vi "BRig_RT__Case_Exp__State_WrongOrTimeout_Pre__v10.vi"(0 "input_dataCurrent":u16[](array[numeric]), 5 "input_WorTO":bool, 7 "input_dataBlock":u16[][](array[numeric]), 9 "input_dataTrial":u16[][](array[numeric]), 11 "input_dataExp":u16[](array[numeric])) -> (1 "output_BTPR":bool, 2 "output_T2R":bool, 3 "output_T2R_or_BTPR":u16, 4 "output_dataCurrent":u16[](array[numeric]), 8 "output_dataBlock":u16[][](array[numeric]), 10 "output_dataTrial":u16[][](array[numeric]), 12 "output_BTPRavg":dbl, 13 "output_T2Ravg":dbl, 14 "output_R(F)_or_L(T)":bool, 15 "output_haveNewAvg":bool)   [LabVIEW 2014]
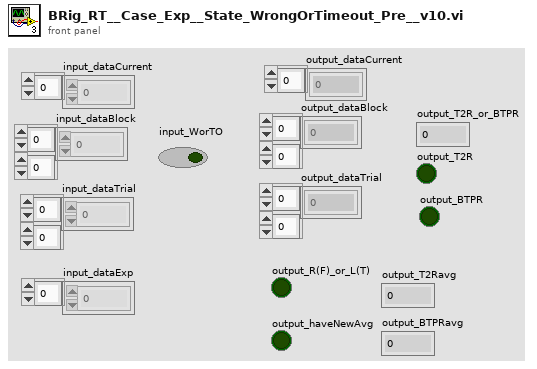
[diagram p1: front panel]
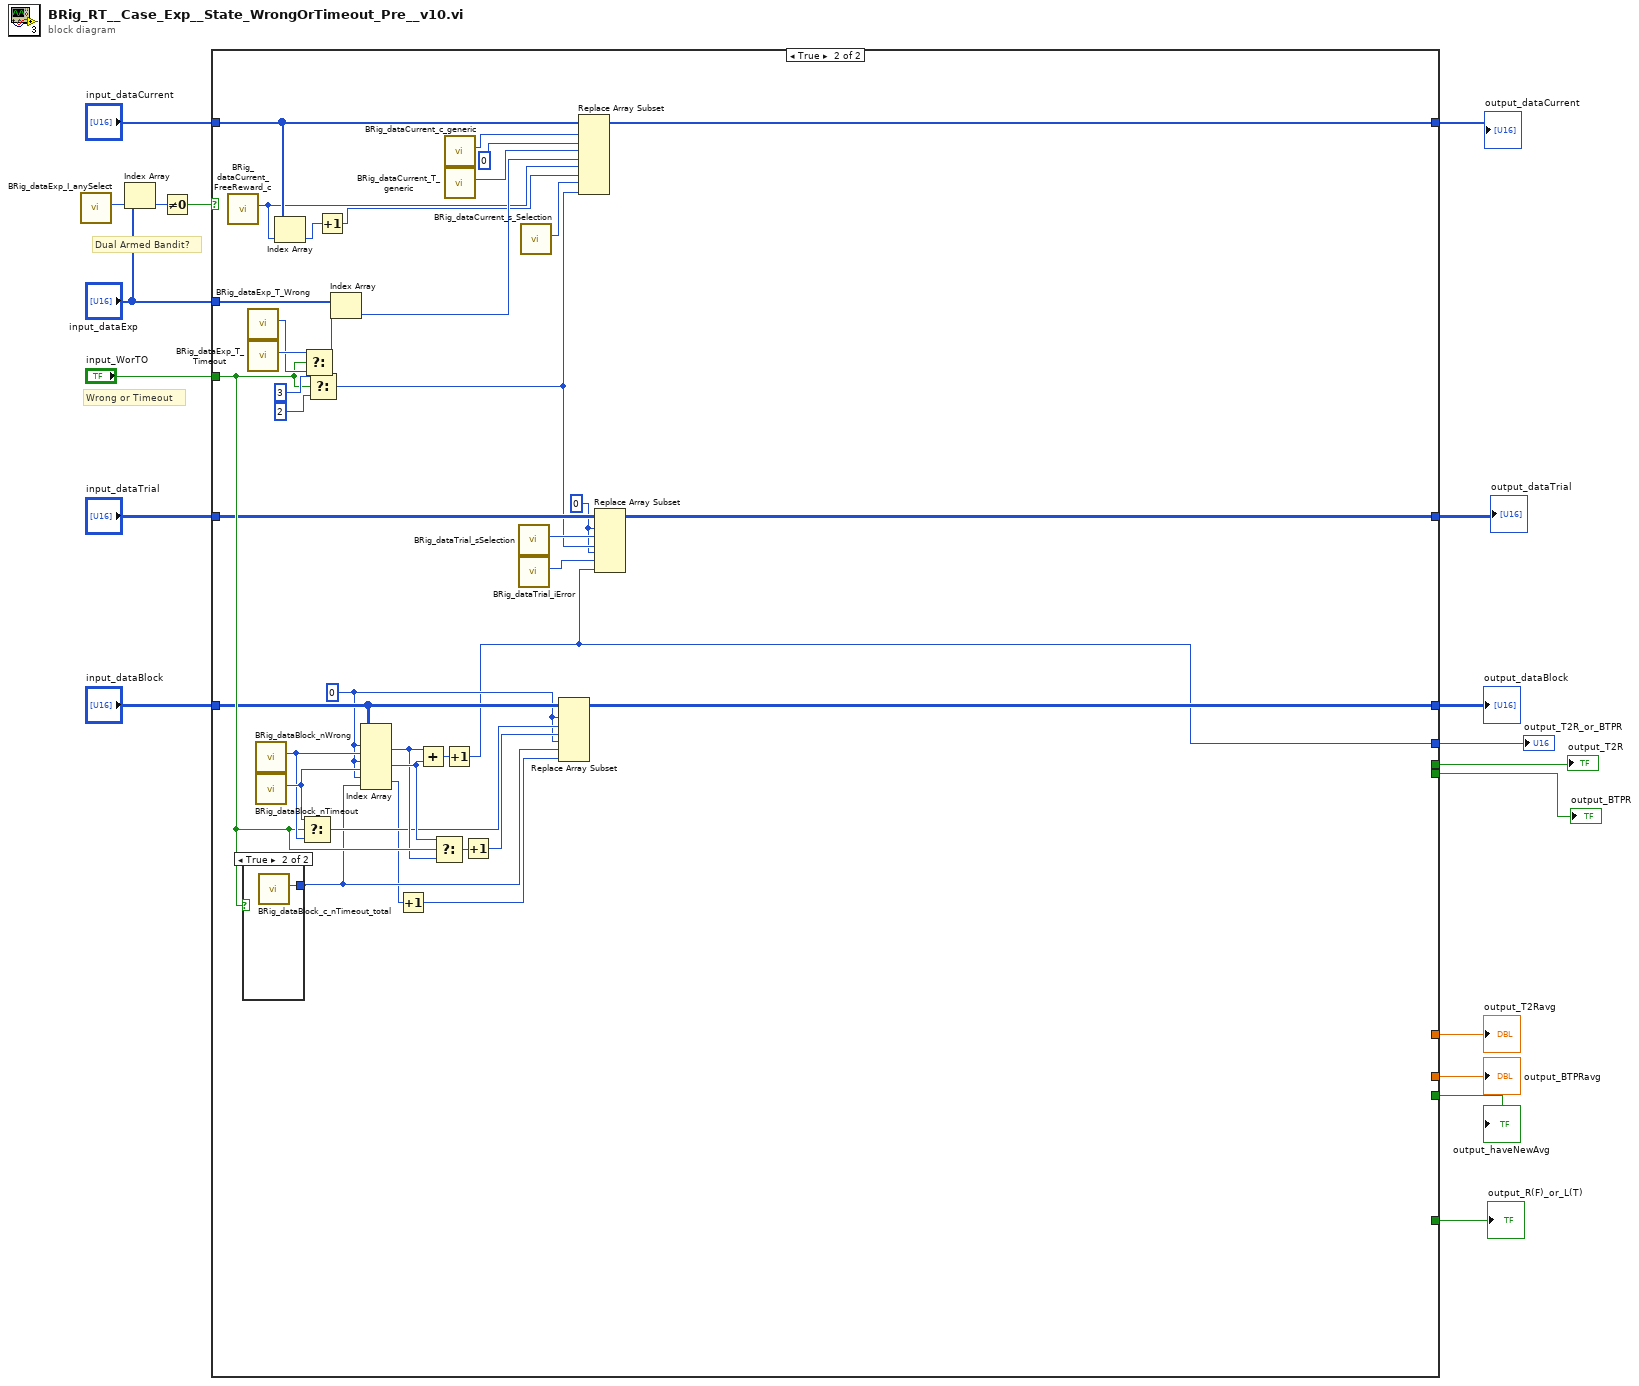
[diagram p0: block diagram]
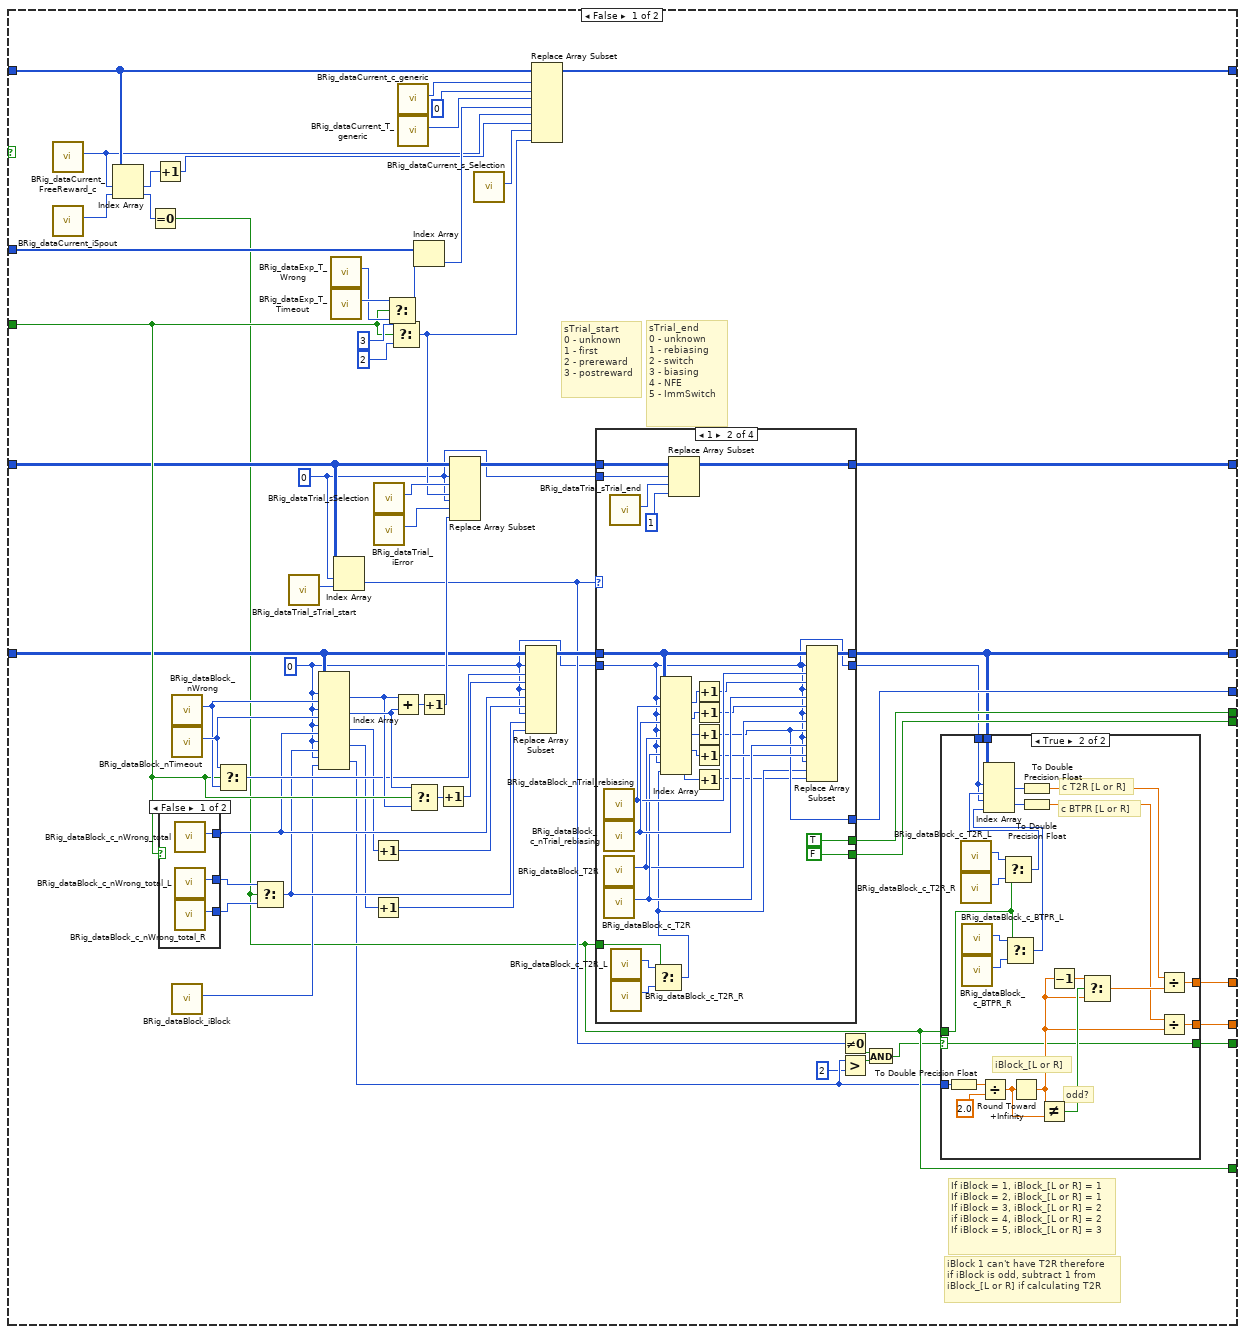
[diagram p2: hidden frame]
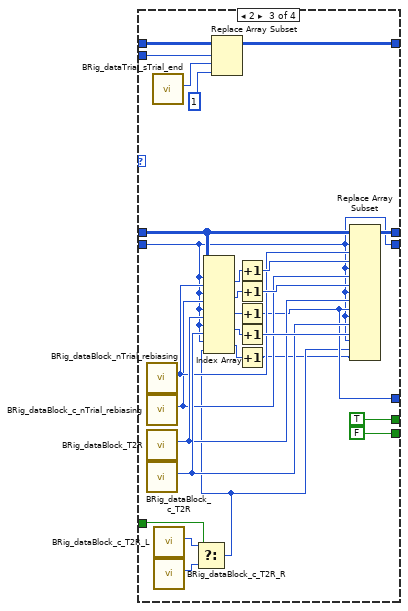
[diagram p5: hidden frame]
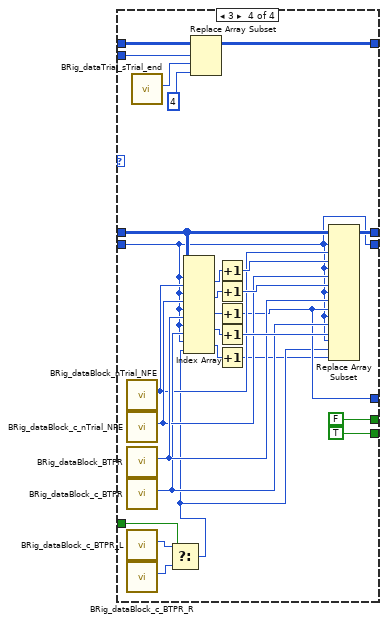
[diagram p6: hidden frame]
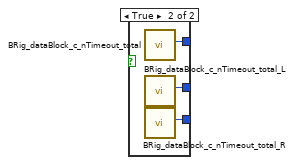
[diagram p7: hidden frame]
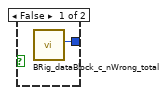
[diagram p8: hidden frame]
diagram:
  # "Wrong or Timeout"
  # "Dual Armed Bandit?"
  n1 = call "BRig_dataExp_I_anySelect.vi"() -> ("output_I_anySelect"=w5:i32)  [unwired: 11 in]
  n2 = Index Array(array="input_dataExp", index=w5) -> (element=w4:u16)
  n3 = Not Equal To 0?(x=w4) -> (x != 0?=w2:bool)
  n4 = case shown="True" w2 {
    tunnel: [w81 w236] -> w18
    tunnel: "input_dataCurrent" -> [w77 w232]
    tunnel: "input_dataExp" -> [w76 w231]
    tunnel: "input_WorTO" -> [w61 w219]
    tunnel: "input_dataBlock" -> [w57 w215]
    tunnel: "input_dataTrial" -> [w47 w209]
    tunnel: [w44 w202] -> w1
    tunnel: [w38 w199] -> w13
    tunnel: [w37 _] -> w12
    tunnel: [w36 _] -> w11
    tunnel: [w29 _] -> w10
    tunnel: [w28 w201] -> w9
    tunnel: [w26 _] -> w8
    tunnel: [w25 _] -> w7
    tunnel: [w24 _] -> w6
    frame False {
      w32 = 0
      w33 = 0
      # "iBlock 1 can't have T2R therefore\nif iBlock is odd, subtract 1 from\niBlock_[L or R] if calculating T2R"
      # "If iBlock = 1, iBlock_[L or R] = 1\nIf iBlock = 2, iBlock_[L or R] = 1\nIf iBlock = 3, iBlock_[L or R] = 2\nif iBlock = 4, iBlock_[L or R] = 2\nIf iBlock = 5, iBlock_[L or R] = 3"
      # "sTrial_end\n0 - unknown\n1 - rebiasing\n2 - switch\n3 - biasing\n4 - NFE\n5 - ImmSwitch"
      # "sTrial_start\n0 - unknown\n1 - first\n2 - prereward\n3 - postreward"
      n5 = call "BRig_dataCurrent_FreeReward_c.vi"() -> ("output_FreeReward_c"=w42:i32)  [unwired: 11 in]
      n6 = call "BRig_dataCurrent_iSpout.vi"() -> ("output_iSpout"=w31:i32)  [unwired: 11 in]
      n7 = Index Array(array=w77, index #1=w42, index #2=w31) -> (element #1=w43:u16, element #2=w30:u16)
      n8 = Equal To 0?(x=w30) -> (x = 0?=w29:bool)
      n9 = Increment(x=w43) -> (x+1=w41:u16)
      n10 = case shown="False" w61 {
        tunnel: [w195 w198] -> w54
        tunnel: [w194 w197] -> w67
        tunnel: [w193 w196] -> w66
        frame False {
          n11 = call "BRig_dataBlock_c_nWrong_total.vi"() -> ("output_c_nWrong_total"=w195:i32)  [unwired: 11 in]
          n12 = call "BRig_dataBlock_c_nWrong_total_L.vi"() -> ("output_c_nWrong_total_L"=w194:i32)  [unwired: 11 in]
          n13 = call "BRig_dataBlock_c_nWrong_total_R.vi"() -> ("output_c_nWrong_total_R"=w193:i32)  [unwired: 11 in]
        }
        frame True {
          n14 = call "BRig_dataBlock_c_nTimeout_total.vi"() -> ("output_c_nTimeout_total"=w198:i32)  [unwired: 11 in]
          n15 = call "BRig_dataBlock_c_nTimeout_total_L.vi"() -> ("output_c_nTimeout_total_L"=w197:i32)  [unwired: 11 in]
          n16 = call "BRig_dataBlock_c_nTimeout_total_R.vi"() -> ("output_c_nTimeout_total_R"=w196:i32)  [unwired: 11 in]
        }
      }
      n17 = call "BRig_dataBlock_nWrong.vi"() -> ("output_nWrong"=w62:i32)  [unwired: 11 in]
      n18 = call "BRig_dataBlock_nTimeout.vi"() -> ("output_nTimeout"=w63:i32)  [unwired: 11 in]
      n19 = call "BRig_dataBlock_iBlock.vi"() -> ("output_iBlock"=w35:i32)  [unwired: 11 in]
      n20 = Select(t=w63, s=w61, f=w62) -> (s? t:f=w56:i32)
      n21 = Select(t=w67, s=w29, f=w66) -> (s? t:f=w53:i32)
      n22 = call "BRig_dataTrial_sTrial_start.vi"() -> ("output_sTrial_start"=w48:i32)  [unwired: 11 in]
      n23 = Index Array(array=w57, index (row) #1=w32, index (col) #1=w62, index (row) #2=w32, index (col) #2=w63, index (row) #3=w32, index (col) #3=w54, index (row) #4=w32, index (col) #4=w53, index (row) #5=w32, index (col) #5=w35) -> (element #1=w59:u16, element #2=w60:u16, element #3=w52:u16, element #4=w51:u16, element #5=w23:u16)
      n24 = call "BRig_dataExp_T_Wrong.vi"() -> ("output_T_Wrong"=w73:i32)  [unwired: 11 in]
      n25 = call "BRig_dataExp_T_Timeout.vi"() -> ("output_T_Timeout"=w74:i32)  [unwired: 11 in]
      n26 = Index Array(array=w47, index (row)=w33, index (col)=w48) -> (element=w34:u16)
      n27 = Increment(x=w52) -> (x+1=w50:u16)
      n28 = Increment(x=w51) -> (x+1=w49:u16)
      n29 = call "BRig_dataTrial_sSelection.vi"() -> ("output_sSelection"=w69:i32)  [unwired: 11 in]
      n30 = call "BRig_dataTrial_iError.vi"() -> ("output_iError"=w68:i32)  [unwired: 11 in]
      n31 = Select(t=w74, s=w61, f=w73) -> (s? t:f=w75:i32)
      n32 = Select(t=u16 3 ("new element/subarray"), s=w61, f=u16 2 ("new element/subarray")) -> (s? t:f=w39:u16)
      n33 = Add(x=w59, y=w60) -> (x+y=w65:u16)
      n34 = call "BRig_dataCurrent_c_generic.vi"() -> ("output_count_generic"=w80:i32)  [unwired: 11 in]
      n35 = call "BRig_dataCurrent_T_generic.vi"() -> ("output_T_generic"=w79:i32)  [unwired: 11 in]
      n36 = Select(t=w60, s=w61, f=w59) -> (s? t:f=w58:u16)
      n37 = Index Array(array=w76, index=w75) -> (element=w72:u16)
      n38 = Increment(x=w65) -> (x+1=w64:u16)
      n39 = Increment(x=w58) -> (x+1=w55:u16)
      n40 = Replace Array Subset(array=w47, new element #1=w39, index (row) #1=w33, index (col) #1=w69, new element #2=w64, index (row) #2=w33, index (col) #2=w68) -> (w46:u16[][])
      n41 = call "BRig_dataCurrent_s_Selection.vi"() -> ("output_s_Selection"=w40:i32)  [unwired: 11 in]
      n42 = Replace Array Subset(array=w57, new element #1=w55, index (row) #1=w32, index (col) #1=w56, new element #2=w50, index (row) #2=w32, index (col) #2=w54, new element #3=w49, index (row) #3=w32, index (col) #3=w53) -> (w45:u16[][])
      n43 = Replace Array Subset(array=w77, new element #1=u16 0 ("new element/subarray"), index #1=w80, new element #2=w72, index #2=w79, new element #3=w41, index #3=w42, new element #4=w39, index #4=w40) -> (w81:u16[])
      n44 = case shown="1" w34 {
        tunnel: w46 -> [w108 w136 w164 w192]
        tunnel: w33 -> [_ w134 w162 w190]
        tunnel: [w108 w135 w163 w191] -> w44
        tunnel: w45 -> [w107 w125 w148 w180]
        tunnel: [w107 w124 w147 w179] -> w28
        tunnel: w32 -> [w106 w109 w137 w165]
        tunnel: [_ w116 w146 w172] -> w38
        tunnel: [_ TRUE TRUE FALSE] -> w37
        tunnel: [_ FALSE FALSE TRUE] -> w36
        tunnel: w29 -> [_ w115 w139 w171]
        tunnel: [w106 w109 w137 w165] -> w27
        frame 0, Default {
        }
        frame 1 {
          n45 = call "BRig_dataBlock_nTrial_rebiasing.vi"() -> ("output_nTrial_rebiasing"=w130:i32)  [unwired: 11 in]
          n46 = call "BRig_dataBlock_c_nTrial_rebiasing.vi"() -> ("output_c_nTrial_rebiasing"=w131:i32)  [unwired: 11 in]
          n47 = call "BRig_dataBlock_T2R.vi"() -> ("output_T2R"=w119:i32)  [unwired: 11 in]
          n48 = call "BRig_dataBlock_c_T2R.vi"() -> ("output_c_T2R"=w121:i32)  [unwired: 11 in]
          n49 = call "BRig_dataTrial_sTrial_end.vi"() -> ("output_sTrial_end"=w133:i32)  [unwired: 11 in]
          n50 = call "BRig_dataBlock_c_T2R_L.vi"() -> ("output_c_T2R_L"=w114:i32)  [unwired: 11 in]
          n51 = call "BRig_dataBlock_c_T2R_R.vi"() -> ("output_c_T2R_R"=w113:i32)  [unwired: 11 in]
          n52 = Select(t=w114, s=w115, f=w113) -> (s? t:f=w111:i32)
          n53 = Index Array(array=w125, index (row) #1=w109, index (col) #1=w130, index (row) #2=w109, index (col) #2=w131, index (row) #3=w109, index (col) #3=w119, index (row) #4=w109, index (col) #4=w121, index (row) #5=w109, index (col) #5=w111) -> (element #1=w129:u16, element #2=w127:u16, element #3=w123:u16, element #4=w122:u16, element #5=w112:u16)
          n54 = Replace Array Subset(array=w136, new element=u16 1 ("new element/subarray"), index (row)=w134, index (col)=w133) -> (w135:u16[][])
          n55 = Increment(x=w129) -> (x+1=w128:u16)
          n56 = Increment(x=w127) -> (x+1=w126:u16)
          n57 = Increment(x=w123) -> (x+1=w116:u16)
          n58 = Increment(x=w122) -> (x+1=w120:u16)
          n59 = Increment(x=w112) -> (x+1=w110:u16)
          n60 = Replace Array Subset(array=w125, new element #1=w128, index (row) #1=w109, index (col) #1=w130, new element #2=w126, index (row) #2=w109, index (col) #2=w131, new element #3=w116, index (row) #3=w109, index (col) #3=w119, new element #4=w120, index (row) #4=w109, index (col) #4=w121, new element #5=w110, index (row) #5=w109, index (col) #5=w111) -> (w124:u16[][])
        }
        frame 2 {
          n61 = call "BRig_dataBlock_nTrial_rebiasing.vi"() -> ("output_nTrial_rebiasing"=w150:i32)  [unwired: 11 in]
          n62 = call "BRig_dataBlock_c_nTrial_rebiasing.vi"() -> ("output_c_nTrial_rebiasing"=w149:i32)  [unwired: 11 in]
          n63 = call "BRig_dataBlock_T2R.vi"() -> ("output_T2R"=w157:i32)  [unwired: 11 in]
          n64 = call "BRig_dataBlock_c_T2R.vi"() -> ("output_c_T2R"=w158:i32)  [unwired: 11 in]
          n65 = call "BRig_dataTrial_sTrial_end.vi"() -> ("output_sTrial_end"=w161:i32)  [unwired: 11 in]
          n66 = call "BRig_dataBlock_c_T2R_L.vi"() -> ("output_c_T2R_L"=w143:i32)  [unwired: 11 in]
          n67 = call "BRig_dataBlock_c_T2R_R.vi"() -> ("output_c_T2R_R"=w142:i32)  [unwired: 11 in]
          n68 = Select(t=w143, s=w139, f=w142) -> (s? t:f=w140:i32)
          n69 = Index Array(array=w148, index (row) #1=w137, index (col) #1=w150, index (row) #2=w137, index (col) #2=w149, index (row) #3=w137, index (col) #3=w157, index (row) #4=w137, index (col) #4=w158, index (row) #5=w137, index (col) #5=w140) -> (element #1=w151:u16, element #2=w153:u16, element #3=w155:u16, element #4=w156:u16, element #5=w141:u16)
          n70 = Replace Array Subset(array=w164, new element=u16 1 ("new element/subarray"), index (row)=w162, index (col)=w161) -> (w163:u16[][])
          n71 = Increment(x=w151) -> (x+1=w152:u16)
          n72 = Increment(x=w153) -> (x+1=w154:u16)
          n73 = Increment(x=w155) -> (x+1=w146:u16)
          n74 = Increment(x=w156) -> (x+1=w159:u16)
          n75 = Increment(x=w141) -> (x+1=w138:u16)
          n76 = Replace Array Subset(array=w148, new element #1=w152, index (row) #1=w137, index (col) #1=w150, new element #2=w154, index (row) #2=w137, index (col) #2=w149, new element #3=w146, index (row) #3=w137, index (col) #3=w157, new element #4=w159, index (row) #4=w137, index (col) #4=w158, new element #5=w138, index (row) #5=w137, index (col) #5=w140) -> (w147:u16[][])
        }
        frame 3 {
          n77 = call "BRig_dataBlock_nTrial_NFE.vi"() -> ("output_nTrial_NFE"=w175:i32)  [unwired: 11 in]
          n78 = call "BRig_dataBlock_c_nTrial_NFE.vi"() -> ("output_c_nTrial_NFE"=w177:i32)  [unwired: 11 in]
          n79 = call "BRig_dataBlock_BTPR.vi"() -> ("output_BTPR"=w178:i32)  [unwired: 11 in]
          n80 = call "BRig_dataBlock_c_BTPR.vi"() -> ("output_c_BTPR"=w176:i32)  [unwired: 11 in]
          n81 = call "BRig_dataBlock_c_BTPR_L.vi"() -> ("output_c_BTPR_L"=w170:i32)  [unwired: 11 in]
          n82 = call "BRig_dataBlock_c_BTPR_R.vi"() -> ("output_c_BTPR_R"=w169:i32)  [unwired: 11 in]
          n83 = call "BRig_dataTrial_sTrial_end.vi"() -> ("output_sTrial_end"=w189:i32)  [unwired: 11 in]
          n84 = Select(t=w170, s=w171, f=w169) -> (s? t:f=w167:i32)
          n85 = Index Array(array=w180, index (row) #1=w165, index (col) #1=w175, index (row) #2=w165, index (col) #2=w177, index (row) #3=w165, index (col) #3=w178, index (row) #4=w165, index (col) #4=w176, index (row) #5=w165, index (col) #5=w167) -> (element #1=w181:u16, element #2=w183:u16, element #3=w185:u16, element #4=w186:u16, element #5=w168:u16)
          n86 = Replace Array Subset(array=w192, new element=u16 4 ("new element/subarray"), index (row)=w190, index (col)=w189) -> (w191:u16[][])
          n87 = Increment(x=w181) -> (x+1=w182:u16)
          n88 = Increment(x=w183) -> (x+1=w184:u16)
          n89 = Increment(x=w185) -> (x+1=w172:u16)
          n90 = Increment(x=w186) -> (x+1=w187:u16)
          n91 = Increment(x=w168) -> (x+1=w166:u16)
          n92 = Replace Array Subset(array=w180, new element #1=w182, index (row) #1=w165, index (col) #1=w175, new element #2=w184, index (row) #2=w165, index (col) #2=w177, new element #3=w172, index (row) #3=w165, index (col) #3=w178, new element #4=w187, index (row) #4=w165, index (col) #4=w176, new element #5=w166, index (row) #5=w165, index (col) #5=w167) -> (w179:u16[][])
        }
      }
      n93 = Not Equal To 0?(x=w34) -> (x != 0?=w20:bool)
      n94 = Greater?(x=w23, y=u16 2) -> (0:w21:bool)
      n95 = And(x=w20, y=w21) -> (x .and. y?=w19:bool)
      n96 = case shown="True" w19 {
        selector: w19 -> [_ w82]
        tunnel: w29 -> [_ w97]
        tunnel: w28 -> [_ w100]
        tunnel: w27 -> [_ w99]
        tunnel: w23 -> [_ w93]
        tunnel: [_ w84] -> w26
        tunnel: [_ w83] -> w25
        tunnel: [_ w82] -> w24
        frame False {
        }
        frame True {
          # "c BTPR [L or R]"
          # "c T2R [L or R]"
          # "odd?"
          # "iBlock_[L or R]"
          n97 = To Double Precision Float(number=w93) -> (double precision float=w96:dbl)
          n98 = call "BRig_dataBlock_c_T2R_L.vi"() -> ("output_c_T2R_L"=w104:i32)  [unwired: 11 in]
          n99 = call "BRig_dataBlock_c_T2R_R.vi"() -> ("output_c_T2R_R"=w105:i32)  [unwired: 11 in]
          n100 = call "BRig_dataBlock_c_BTPR_L.vi"() -> ("output_c_BTPR_L"=w102:i32)  [unwired: 11 in]
          n101 = call "BRig_dataBlock_c_BTPR_R.vi"() -> ("output_c_BTPR_R"=w103:i32)  [unwired: 11 in]
          n102 = Divide(x=w96, y=2.0) -> (x/y=w94:dbl)
          n103 = Select(t=w104, s=w97, f=w105) -> (s? t:f=w101:i32)
          n104 = Select(t=w102, s=w97, f=w103) -> (s? t:f=w98:i32)
          n105 = Index Array(array=w100, index (row) #1=w99, index (col) #1=w101, index (row) #2=w99, index (col) #2=w98) -> (element #1=w88:u16, element #2=w89:u16)
          n106 = Round Toward +Infinity(x=w94) -> (ceil(x): smallest int >= x=w87:dbl)
          n107 = To Double Precision Float(number=w88) -> (double precision float=w86:dbl)
          n108 = To Double Precision Float(number=w89) -> (double precision float=w85:dbl)
          n109 = Not Equal?(x=w87, y=w94) -> (x != y?=w91:bool)
          n110 = Decrement(x=w87) -> (x-1=w92:dbl)
          n111 = Select(t=w92, s=w91, f=w87) -> (s? t:f=w90:dbl)
          n112 = Divide(x=w86, y=w90) -> (x/y=w84:dbl)
          n113 = Divide(x=w85, y=w87) -> (x/y=w83:dbl)
        }
      }
    }
    frame True {
      w200 = 0
      w203 = 0
      n114 = call "BRig_dataCurrent_FreeReward_c.vi"() -> ("output_FreeReward_c"=w207:i32)  [unwired: 11 in]
      n115 = case shown="True" w219 {
        tunnel: [w237 w238] -> w212
        frame False {
          n116 = call "BRig_dataBlock_c_nWrong_total.vi"() -> ("output_c_nWrong_total"=w237:i32)  [unwired: 11 in]
        }
        frame True {
          n117 = call "BRig_dataBlock_c_nTimeout_total.vi"() -> ("output_c_nTimeout_total"=w238:i32)  [unwired: 11 in]
        }
      }
      n118 = call "BRig_dataExp_T_Wrong.vi"() -> ("output_T_Wrong"=w228:i32)  [unwired: 11 in]
      n119 = call "BRig_dataExp_T_Timeout.vi"() -> ("output_T_Timeout"=w229:i32)  [unwired: 11 in]
      n120 = call "BRig_dataBlock_nWrong.vi"() -> ("output_nWrong"=w220:i32)  [unwired: 11 in]
      n121 = call "BRig_dataBlock_nTimeout.vi"() -> ("output_nTimeout"=w221:i32)  [unwired: 11 in]
      n122 = Index Array(array=w232, index=w207) -> (element=w208:u16)
      n123 = Select(t=w221, s=w219, f=w220) -> (s? t:f=w214:i32)
      n124 = Select(t=w229, s=w219, f=w228) -> (s? t:f=w230:i32)
      n125 = Select(t=u16 3 ("new element/subarray"), s=w219, f=u16 2 ("new element/subarray")) -> (s? t:f=w204:u16)
      n126 = Increment(x=w208) -> (x+1=w206:u16)
      n127 = Index Array(array=w231, index=w230) -> (element=w227:u16)
      n128 = Index Array(array=w215, index (row) #1=w200, index (col) #1=w220, index (row) #2=w200, index (col) #2=w221, index (row) #3=w200, index (col) #3=w212) -> (element #1=w217:u16, element #2=w218:u16, element #3=w211:u16)
      n129 = Increment(x=w211) -> (x+1=w210:u16)
      n130 = Add(x=w217, y=w218) -> (x+y=w222:u16)
      n131 = Select(t=w218, s=w219, f=w217) -> (s? t:f=w216:u16)
      n132 = Increment(x=w222) -> (x+1=w199:u16)
      n133 = call "BRig_dataCurrent_c_generic.vi"() -> ("output_count_generic"=w235:i32)  [unwired: 11 in]
      n134 = call "BRig_dataCurrent_T_generic.vi"() -> ("output_T_generic"=w234:i32)  [unwired: 11 in]
      n135 = Increment(x=w216) -> (x+1=w213:u16)
      n136 = call "BRig_dataTrial_sSelection.vi"() -> ("output_sSelection"=w224:i32)  [unwired: 11 in]
      n137 = call "BRig_dataTrial_iError.vi"() -> ("output_iError"=w223:i32)  [unwired: 11 in]
      n138 = call "BRig_dataCurrent_s_Selection.vi"() -> ("output_s_Selection"=w205:i32)  [unwired: 11 in]
      n139 = Replace Array Subset(array=w215, new element #1=w213, index (row) #1=w200, index (col) #1=w214, new element #2=w210, index (row) #2=w200, index (col) #2=w212) -> (w201:u16[][])
      n140 = Replace Array Subset(array=w232, new element #1=u16 0 ("new element/subarray"), index #1=w235, new element #2=w227, index #2=w234, new element #3=w206, index #3=w207, new element #4=w204, index #4=w205) -> (w236:u16[])
      n141 = Replace Array Subset(array=w209, new element #1=w204, index (row) #1=w203, index (col) #1=w224, new element #2=w199, index (row) #2=w203, index (col) #2=w223) -> (w202:u16[][])
    }
  }
  "output_dataCurrent" <- w18
  "output_dataBlock" <- w9
  "output_dataTrial" <- w1
  "output_T2R_or_BTPR" <- w13
  "output_T2R" <- w12
  "output_BTPR" <- w11
  "output_R(F)_or_L(T)" <- w10
  "output_T2Ravg" <- w8
  "output_BTPRavg" <- w7
  "output_haveNewAvg" <- w6
